vi "tcsWEP_getSample_loopTimeMs.vi"(8 "error in (no error)":errorcluster, 11 "loopTimeMs_Ctl":T1) -> (0 "error out":errorcluster, 2 "function return":i32, 3 "loopTimeMs_Ctl out":T1)   [LabVIEW 2016, in "SALLV_tcsWEP.lvlib"]
doc: "int tcsWEP_shm_getSample_loopTimeMsLV(tcsWEP_loopTimeMsLV *loopTimeMs_Ctl );"
uses:
  SALLV_tcsWEP.lvlib
  DataTypes/loopTimeMs.ctl
  SALLV_tcsWEP.so
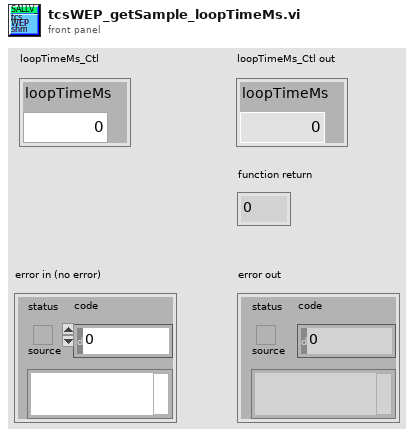
[diagram p1: front panel]
types:
  T1 = typedef "SALLV_tcsWEP.lvlib/loopTimeMs.ctl" = cluster{"loopTimeMs":dbl}
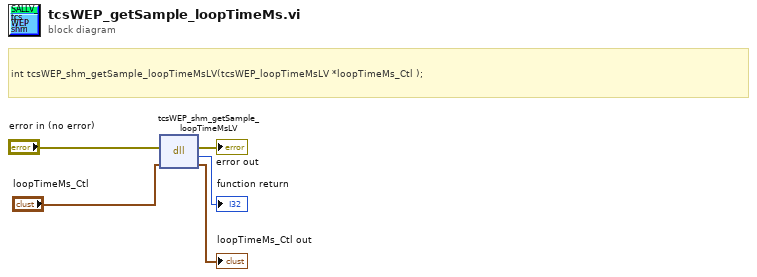
[diagram p0: block diagram]
diagram:
  # "int tcsWEP_shm_getSample_loopTimeMsLV(tcsWEP_loopTimeMsLV *loopTimeMs_Ctl );"
  n1 = dll-call lib="home/ttsai/Documents/salAPI/SALLV_tcsWEP.*" fn="tcsWEP_shm_getSample_loopTimeMsLV"(error in="error in (no error)", "loopTimeMs_Ctl"="loopTimeMs_Ctl") -> (error out=→"error out":errorcluster, →"function return":i32, "loopTimeMs_Ctl"=→"loopTimeMs_Ctl out":T1)  [unwired: 2 in, 1 out]
